vi "Read HH Chans Used.vi"(8 "error in (no error)":errorcluster, 10 "HH Chans Used":i32[](array[numeric]), 11 "DCM-DSI-HW in":refnum<class "DCM-DSI.lvclass">) -> (0 "error out":errorcluster, 3 "DCM-DSI-HW out":refnum<class "DCM-DSI.lvclass">)   [LabVIEW 2016, in "DCM-DSI.lvclass"]
uses:
  DCM-DSI.lvclass
  DCM-DSI.lvclass/DCM-DSI.ctl
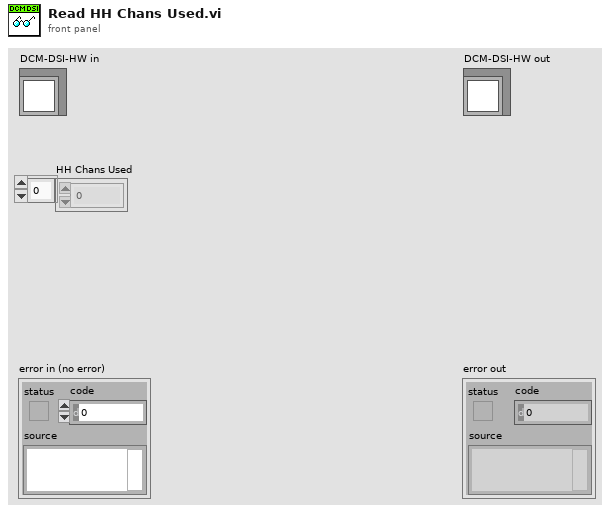
[diagram p1: front panel]
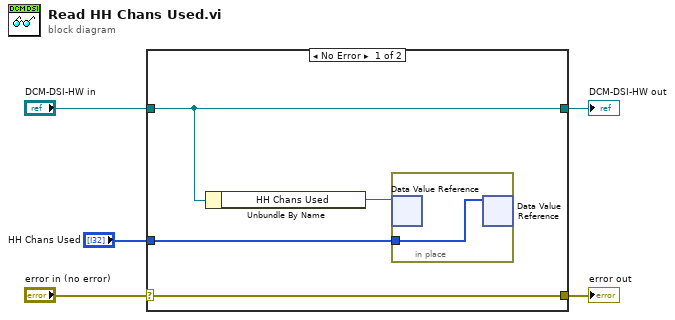
[diagram p0: block diagram]
diagram:
  n1 = case shown="No Error" "error in (no error)" {
    selector: "error in (no error)" -> [w9 w12]
    tunnel: [w9 w12] -> w4
    tunnel: [w7 w11] -> w2
    tunnel: "DCM-DSI-HW in" -> [w7 w11]
    tunnel: "HH Chans Used" -> [w6 _]
    frame No Error {
      n2 = Unbundle By Name(w7) -> ("HH Chans Used"=w8:refnum<data-value>)
      n3 = in-place {
        in-place-border: w6 -> [w10]
        n4 = in-place-dvr #1(w8) -> ()  [unwired: 2 out]
        n5 = in-place-dvr #1(w10) -> ()  [unwired: 2 out]
      }
    }
    frame Error {
    }
  }
  "error out" <- w4
  "DCM-DSI-HW out" <- w2
